vi "Experiment header-Overwrite values.vi"(10 "All header parameters in":T1={"LOGIN"={"User"="", "Profile"="", "Software Version"="", "Experiment Date Time"=timestamp(0 s since 1904-01-01)}, "GLOBAL PARAMETERS"={"MicroscopeID"="", "Microscope Type"="", "Objective"="", "Field of View (um)"=0.0, "Fill time (us)"=0.0, "Experiment Type"=enum."In vivo", "Stimuli Trigger"=FALSE, "Speed Logging"=FALSE}, "IMAGING MODES"={"Time Series"=FALSE, "Motor Zstack"=FALSE, "AOL Zstack"=FALSE, "Functional Imaging"=FALSE, "Volume Imaging"=FALSE}, "TIME SERIES"={"Basic Image meta data"={"Wavelength (nm)"=0.0, "# averaged frames"=0.0, "laser power (%)"=0.0, "Pockels"=0.0, "pixel dwell time (us)"=0.0, "pmt 1"=0.0, "pmt 2"=0.0, "back apperture"=0.0, "zoom"=0.0, "field of view"=0.0, "Frame Size"=0, "AOL x centre"=0.0, "AOL y centre"=0.0, "Stage x position"=0.0, "Stage y position"=0.0, "Stage z position"=0.0}, "AOL z"=0.0}, "MOTOR Z-STACK "={"Hdr Basic Image meta data"={"Wavelength (nm)"=0.0, "# averaged frames"=0.0, "laser power (%)"=0.0, "Pockels"=0.0, "pixel dwell time (us)"=0.0, "pmt 1"=0.0, "pmt 2"=0.0, "back apperture"=0.0, "zoom"=0.0, "field of view"=0.0, "Frame Size"=0, "AOL x centre"=0.0, "AOL y centre"=0.0, "Stage x position"=0.0, "Stage y position"=0.0, "Stage z position"=0.0}, "Z Start"=0.0, "Z Stop"=0.0, "No of Planes"=0, "Laser Power (%) at Z Start"=0.0, "Laser Power (%) at Z Stop"=0.0}, "AOL Z-STACK"={"Hdr Basic Image meta data"={"Wavelength (nm)"=0.0, "# averaged frames"=0.0, "laser power (%)"=0.0, "Pockels"=0.0, "pixel dwell time (us)"=0.0, "pmt 1"=0.0, "pmt 2"=0.0, "back apperture"=0.0, "zoom"=0.0, "field of view"=0.0, "Frame Size"=0, "AOL x centre"=0.0, "AOL y centre"=0.0, "Stage x position"=0.0, "Stage y position"=0.0, "Stage z position"=0.0}, "Z Start"=0.0, "Z Stop"=0.0, "No of Planes"=0, "Laser Power (%) at Z Start"=0.0, "Laser Power (%) at Z Stop"=0.0}, "FUNCTIONAL IMAGING"={"Functional Mode"=enum."Point", "Variable Length"=FALSE, "Variable Resolution"=FALSE, "Pockels Modulation"=FALSE, "Stimuli Trigger"=FALSE, "Cool down enabled"=FALSE, "AOL Mode"=enum."Raster", "Plane Mode"=0, "Miniscan Dwell time per pixel (us)"=0.0, "poi dwell time"=0.0, "Number of trials"=0.0, "Number of cycles"=0.0, "Number of pois"=0.0, "Number of miniscans"=0.0, "Number of pixels in miniscan"=0.0, "Rectangle ROI length"=0.0, "Rectangle ROI height"=0.0, "Frame rate (fps)"=0.0, "Acquisition Length"=0.0, "video length (sec)"=0.0, "Stimuli delay (sec)"=0.0, "Cool down time (sec)"=0.0, "Basic Image meta data"={"Wavelength (nm)"=0.0, "# averaged frames"=0.0, "laser power (%)"=0.0, "Pockels"=0.0, "pixel dwell time (us)"=0.0, "pmt 1"=0.0, "pmt 2"=0.0, "back apperture"=0.0, "zoom"=0.0, "field of view"=0.0, "Frame Size"=0, "AOL x centre"=0.0, "AOL y centre"=0.0, "Stage x position"=0.0, "Stage y position"=0.0, "Stage z position"=0.0}, "Z Start (um)"=0.0, "Z Stop (um)"=0.0}, "VOLUME IMAGING"={"Functional Mode"=enum."Point", "Variable Length"=FALSE, "Variable Resolution"=FALSE, "Pockels Modulation"=FALSE, "Stimuli Trigger"=FALSE, "Cool down enabled"=FALSE, "AOL Mode"=enum."Raster", "Plane Mode"=0, "Miniscan Dwell time per pixel (us)"=0.0, "poi dwell time"=0.0, "Number of trials"=0.0, "Number of cycles"=0.0, "Number of pois"=0.0, "Number of miniscans"=0.0, "Number of pixels in miniscan"=0.0, "Rectangle ROI length"=0.0, "Rectangle ROI height"=0.0, "Frame rate (fps)"=0.0, "Acquisition Length"=0.0, "video length (sec)"=0.0, "Stimuli delay (sec)"=0.0, "Cool down time (sec)"=0.0, "Basic Image meta data"={"Wavelength (nm)"=0.0, "# averaged frames"=0.0, "laser power (%)"=0.0, "Pockels"=0.0, "pixel dwell time (us)"=0.0, "pmt 1"=0.0, "pmt 2"=0.0, "back apperture"=0.0, "zoom"=0.0, "field of view"=0.0, "Frame Size"=0, "AOL x centre"=0.0, "AOL y centre"=0.0, "Stage x position"=0.0, "Stage y position"=0.0, "Stage z position"=0.0}, "Z Start (um)"=0.0, "Z Stop (um)"=0.0}, "MOVEMENT CORRECTION"={"Movement Correction"=FALSE, "Axial Reference"=FALSE, "Reference Source"=enum."Green channel", "Full Frame Size"=0.0, "Reference Field of View"=0.0, "Reference Zoom"=0.0, "Reference dwell time (us)"=0.0, "Reference X Pixels"=0.0, "Reference Y Pixels"=0.0, "Number of Z lines"=0.0, "Size of Z pixels"=0.0, "Axial Pixels"=0.0, "Ignore Z lines"=0.0, "Reference Scan Cycles"=0.0, "Reference Threshold XY"=0.0, "Reference Threshold Z"=0.0, "Reference Average XY"=0.0, "Reference Average Z"=0.0, "Proportional Scale"=0.0, "Integral Scale"=0.0, "Proportional Scale Z"=0.0, "Integral Scale Z"=0.0, "Diff Threshold"=0.0, "Diff Threshold Z"=0.0, "Sliding Average"=FALSE, "Reference count reset enabled"=FALSE, "Scan Interval (ms)"=0.0, "Ref Plot Refresh Rate (ms)"=0.0}, "CALIBRATION"={"Pockels Calibration File"=path "", "Calibration_ini file"=path "", "Setup_ini file"=path ""}, "STATISTICS"={"Z-stack duration (sec)"=0.0, "Number of acquired data-points"=0.0, "Acquisition time (ms)"=0.0, "Number of acquired frames"=0.0, "Intertrial times"=[]}, "BIOLOGY INFORMATION"={"Animal Code or Name"="", "Animal DoB"="", "Animal Age"="", "Animal Sex"="", "Animal Weight"="", "Date of Injection"="", "Date of Implant"="", "Site of Injection"="", "Animal Ear Notch"="", "AAV constructs"="", "Genetic background"="", "Optical reporter"="", "Region of brain imaged"="", "Other \ncomments"=""}, "Calibration Data"={"Objective Name"="", "Calibration Wavelength"=0.0, "Sum X"=0.0, "Sum Y"=0.0, "Diff X"=0.0, "Diff Y"=0.0, "Distortion Correction"=0.0, " Z norm to um Scaling"=0.0, " X norm to um Scaling"=0.0}, "Parameter Sweep Settings"={"Parameter Sweep Steps"={"MB Sep Start"=0.0, "MB Sep Stop"=0.25, "MB Sep Step"=1.0}, "Parameter Sweep"=enum."Dwell Time [us]", "# Sw. Planes"=0, "Basic image meta-data"={"Wavelength (nm)"=0.0, "# averaged frames"=0.0, "laser power (%)"=0.0, "Pockels"=0.0, "pixel dwell time (us)"=0.0, "pmt 1"=0.0, "pmt 2"=0.0, "back apperture"=0.0, "zoom"=0.0, "field of view"=0.0, "Frame Size"=200, "AOL x centre"=0.0, "AOL y centre"=0.0, "Stage x position"=0.0, "Stage y position"=0.0, "Stage z position"=0.0}}} {"Parameter Sweep Settings"."Basic image meta-data"."Frame Size" items=["100X100"=100, "128X128"=128, "200X200"=200, "256X256"=256, "512X512"=512, "1024x1024"=1024, "2048x2048"=2048]; "VOLUME IMAGING"."Plane Mode" items=["XY Plane", "XZ Plane", "YZ Plane", "arbitraryplane"]; "VOLUME IMAGING"."Basic Image meta data"."Frame Size" items=["100X100"=100, "128X128"=128, "200X200"=200, "256X256"=256, "512X512"=512, "1024x1024"=1024, "2048x2048"=2048]; "AOL Z-STACK"."Hdr Basic Image meta data"."Frame Size" items=["100X100"=100, "128X128"=128, "200X200"=200, "256X256"=256, "512X512"=512, "1024x1024"=1024, "2048x2048"=2048]; "MOTOR Z-STACK"."Hdr Basic Image meta data"."Frame Size" items=["100X100"=100, "128X128"=128, "200X200"=200, "256X256"=256, "512X512"=512, "1024x1024"=1024, "2048x2048"=2048]; "FUNCTIONAL IMAGING"."Plane Mode" items=["XY Plane", "XZ Plane", "YZ Plane", "arbitraryplane"]; "FUNCTIONAL IMAGING"."Basic Image meta data"."Frame Size" items=["100X100"=100, "128X128"=128, "200X200"=200, "256X256"=256, "512X512"=512, "1024x1024"=1024, "2048x2048"=2048]; "TIME SERIES"."Basic Image meta data"."Frame Size" items=["100X100"=100, "128X128"=128, "200X200"=200, "256X256"=256, "512X512"=512, "1024x1024"=1024, "2048x2048"=2048]}) -> (2 "All header parameters (FOV converted to um)":T1={"LOGIN"={"User"="", "Profile"="", "Software Version"="", "Experiment Date Time"=timestamp(0 s since 1904-01-01)}, "GLOBAL PARAMETERS"={"MicroscopeID"="", "Microscope Type"="", "Objective"="", "Field of View (um)"=0.0, "Fill time (us)"=0.0, "Experiment Type"=enum."In vivo", "Stimuli Trigger"=FALSE, "Speed Logging"=FALSE}, "IMAGING MODES"={"Time Series"=FALSE, "Motor Zstack"=FALSE, "AOL Zstack"=FALSE, "Functional Imaging"=FALSE, "Volume Imaging"=FALSE}, "TIME SERIES"={"Basic Image meta data"={"Wavelength (nm)"=0.0, "# averaged frames"=0.0, "laser power (%)"=0.0, "Pockels"=0.0, "pixel dwell time (us)"=0.0, "pmt 1"=0.0, "pmt 2"=0.0, "back apperture"=0.0, "zoom"=0.0, "field of view"=0.0, "Frame Size"=0, "AOL x centre"=0.0, "AOL y centre"=0.0, "Stage x position"=0.0, "Stage y position"=0.0, "Stage z position"=0.0}, "AOL z"=0.0}, "MOTOR Z-STACK "={"Hdr Basic Image meta data"={"Wavelength (nm)"=0.0, "# averaged frames"=0.0, "laser power (%)"=0.0, "Pockels"=0.0, "pixel dwell time (us)"=0.0, "pmt 1"=0.0, "pmt 2"=0.0, "back apperture"=0.0, "zoom"=0.0, "field of view"=0.0, "Frame Size"=0, "AOL x centre"=0.0, "AOL y centre"=0.0, "Stage x position"=0.0, "Stage y position"=0.0, "Stage z position"=0.0}, "Z Start"=0.0, "Z Stop"=0.0, "No of Planes"=0, "Laser Power (%) at Z Start"=0.0, "Laser Power (%) at Z Stop"=0.0}, "AOL Z-STACK"={"Hdr Basic Image meta data"={"Wavelength (nm)"=0.0, "# averaged frames"=0.0, "laser power (%)"=0.0, "Pockels"=0.0, "pixel dwell time (us)"=0.0, "pmt 1"=0.0, "pmt 2"=0.0, "back apperture"=0.0, "zoom"=0.0, "field of view"=0.0, "Frame Size"=0, "AOL x centre"=0.0, "AOL y centre"=0.0, "Stage x position"=0.0, "Stage y position"=0.0, "Stage z position"=0.0}, "Z Start"=0.0, "Z Stop"=0.0, "No of Planes"=0, "Laser Power (%) at Z Start"=0.0, "Laser Power (%) at Z Stop"=0.0}, "FUNCTIONAL IMAGING"={"Functional Mode"=enum."Point", "Variable Length"=FALSE, "Variable Resolution"=FALSE, "Pockels Modulation"=FALSE, "Stimuli Trigger"=FALSE, "Cool down enabled"=FALSE, "AOL Mode"=enum."Raster", "Plane Mode"=0, "Miniscan Dwell time per pixel (us)"=0.0, "poi dwell time"=0.0, "Number of trials"=0.0, "Number of cycles"=0.0, "Number of pois"=0.0, "Number of miniscans"=0.0, "Number of pixels in miniscan"=0.0, "Rectangle ROI length"=0.0, "Rectangle ROI height"=0.0, "Frame rate (fps)"=0.0, "Acquisition Length"=0.0, "video length (sec)"=0.0, "Stimuli delay (sec)"=0.0, "Cool down time (sec)"=0.0, "Basic Image meta data"={"Wavelength (nm)"=0.0, "# averaged frames"=0.0, "laser power (%)"=0.0, "Pockels"=0.0, "pixel dwell time (us)"=0.0, "pmt 1"=0.0, "pmt 2"=0.0, "back apperture"=0.0, "zoom"=0.0, "field of view"=0.0, "Frame Size"=0, "AOL x centre"=0.0, "AOL y centre"=0.0, "Stage x position"=0.0, "Stage y position"=0.0, "Stage z position"=0.0}, "Z Start (um)"=0.0, "Z Stop (um)"=0.0}, "VOLUME IMAGING"={"Functional Mode"=enum."Point", "Variable Length"=FALSE, "Variable Resolution"=FALSE, "Pockels Modulation"=FALSE, "Stimuli Trigger"=FALSE, "Cool down enabled"=FALSE, "AOL Mode"=enum."Raster", "Plane Mode"=0, "Miniscan Dwell time per pixel (us)"=0.0, "poi dwell time"=0.0, "Number of trials"=0.0, "Number of cycles"=0.0, "Number of pois"=0.0, "Number of miniscans"=0.0, "Number of pixels in miniscan"=0.0, "Rectangle ROI length"=0.0, "Rectangle ROI height"=0.0, "Frame rate (fps)"=0.0, "Acquisition Length"=0.0, "video length (sec)"=0.0, "Stimuli delay (sec)"=0.0, "Cool down time (sec)"=0.0, "Basic Image meta data"={"Wavelength (nm)"=0.0, "# averaged frames"=0.0, "laser power (%)"=0.0, "Pockels"=0.0, "pixel dwell time (us)"=0.0, "pmt 1"=0.0, "pmt 2"=0.0, "back apperture"=0.0, "zoom"=0.0, "field of view"=0.0, "Frame Size"=0, "AOL x centre"=0.0, "AOL y centre"=0.0, "Stage x position"=0.0, "Stage y position"=0.0, "Stage z position"=0.0}, "Z Start (um)"=0.0, "Z Stop (um)"=0.0}, "MOVEMENT CORRECTION"={"Movement Correction"=FALSE, "Axial Reference"=FALSE, "Reference Source"=enum."Green channel", "Full Frame Size"=0.0, "Reference Field of View"=0.0, "Reference Zoom"=0.0, "Reference dwell time (us)"=0.0, "Reference X Pixels"=0.0, "Reference Y Pixels"=0.0, "Number of Z lines"=0.0, "Size of Z pixels"=0.0, "Axial Pixels"=0.0, "Ignore Z lines"=0.0, "Reference Scan Cycles"=0.0, "Reference Threshold XY"=0.0, "Reference Threshold Z"=0.0, "Reference Average XY"=0.0, "Reference Average Z"=0.0, "Proportional Scale"=0.0, "Integral Scale"=0.0, "Proportional Scale Z"=0.0, "Integral Scale Z"=0.0, "Diff Threshold"=0.0, "Diff Threshold Z"=0.0, "Sliding Average"=FALSE, "Reference count reset enabled"=FALSE, "Scan Interval (ms)"=0.0, "Ref Plot Refresh Rate (ms)"=0.0}, "CALIBRATION"={"Pockels Calibration File"=path "", "Calibration_ini file"=path "", "Setup_ini file"=path ""}, "STATISTICS"={"Z-stack duration (sec)"=0.0, "Number of acquired data-points"=0.0, "Acquisition time (ms)"=0.0, "Number of acquired frames"=0.0, "Intertrial times"=[]}, "BIOLOGY INFORMATION"={"Animal Code or Name"="", "Animal DoB"="", "Animal Age"="", "Animal Sex"="", "Animal Weight"="", "Date of Injection"="", "Date of Implant"="", "Site of Injection"="", "Animal Ear Notch"="", "AAV constructs"="", "Genetic background"="", "Optical reporter"="", "Region of brain imaged"="", "Other \ncomments"=""}, "Calibration Data"={"Objective Name"="", "Calibration Wavelength"=0.0, "Sum X"=0.0, "Sum Y"=0.0, "Diff X"=0.0, "Diff Y"=0.0, "Distortion Correction"=0.0, " Z norm to um Scaling"=0.0, " X norm to um Scaling"=0.0}, "Parameter Sweep Settings"={"Parameter Sweep Steps"={"MB Sep Start"=0.0, "MB Sep Stop"=0.25, "MB Sep Step"=1.0}, "Parameter Sweep"=enum."Dwell Time [us]", "# Sw. Planes"=0, "Basic image meta-data"={"Wavelength (nm)"=0.0, "# averaged frames"=0.0, "laser power (%)"=0.0, "Pockels"=0.0, "pixel dwell time (us)"=0.0, "pmt 1"=0.0, "pmt 2"=0.0, "back apperture"=0.0, "zoom"=0.0, "field of view"=0.0, "Frame Size"=200, "AOL x centre"=0.0, "AOL y centre"=0.0, "Stage x position"=0.0, "Stage y position"=0.0, "Stage z position"=0.0}}} {"Parameter Sweep Settings"."Basic image meta-data"."Frame Size" items=["100X100"=100, "128X128"=128, "200X200"=200, "256X256"=256, "512X512"=512, "1024x1024"=1024, "2048x2048"=2048]; "VOLUME IMAGING"."Plane Mode" items=["XY Plane", "XZ Plane", "YZ Plane", "arbitraryplane"]; "VOLUME IMAGING"."Basic Image meta data"."Frame Size" items=["100X100"=100, "128X128"=128, "200X200"=200, "256X256"=256, "512X512"=512, "1024x1024"=1024, "2048x2048"=2048]; "AOL Z-STACK"."Hdr Basic Image meta data"."Frame Size" items=["100X100"=100, "128X128"=128, "200X200"=200, "256X256"=256, "512X512"=512, "1024x1024"=1024, "2048x2048"=2048]; "MOTOR Z-STACK"."Hdr Basic Image meta data"."Frame Size" items=["100X100"=100, "128X128"=128, "200X200"=200, "256X256"=256, "512X512"=512, "1024x1024"=1024, "2048x2048"=2048]; "FUNCTIONAL IMAGING"."Plane Mode" items=["XY Plane", "XZ Plane", "YZ Plane", "arbitraryplane"]; "FUNCTIONAL IMAGING"."Basic Image meta data"."Frame Size" items=["100X100"=100, "128X128"=128, "200X200"=200, "256X256"=256, "512X512"=512, "1024x1024"=1024, "2048x2048"=2048]; "TIME SERIES"."Basic Image meta data"."Frame Size" items=["100X100"=100, "128X128"=128, "200X200"=200, "256X256"=256, "512X512"=512, "1024x1024"=1024, "2048x2048"=2048]}, 3 "Field of view (um)":dbl)   [LabVIEW 2020]
uses:
  Global Variables/gl_UI Ctrl Refs.vi
  Typedefs/Header subclusters/Header params -Login.ctl
  Misc/Experiment Type.ctl
  Typedefs/Header subclusters/Header params-Global Parameters.ctl
  Typedefs/Header subclusters/Header params-Imaging Modes.ctl
  Typedefs/Header subclusters/Header params-Basic image meta data.ctl
  Typedefs/Header subclusters/Header params-Time Series.ctl
  Typedefs/Header subclusters/Header params-Functional Imaging.ctl
  Typedefs/Reference source.ctl
  Typedefs/Header subclusters/Header params-Movement correction.ctl
  Typedefs/Header subclusters/Header params-Calibration Setup.ctl
  Typedefs/Header subclusters/Header params-statistics.ctl
  Misc/Biology Information.ctl
  Typedefs/Header subclusters/Header params-Motor Z-stack.ctl
  Typedefs/Header subclusters/Header params-AOL Z-stack.ctl
  Typedefs/Header parameters cluster-ALL.ctl
  Typedefs/Frame Size.ctl
  Typedefs/Functional Mode.ctl
  Typedefs/AOL modes.ctl
  Typedefs/Plane Mode.ctl
  Typedefs/Header subclusters/Header params-calibration data.ctl
  Typedefs/Parameter sweep modes.ctl
  Typedefs/Parameter Sweep Steps.ctl
  Typedefs/Header subclusters/Header params-Parameter Sweep.ctl
panel:
  in  "error in (no error)":errorcluster
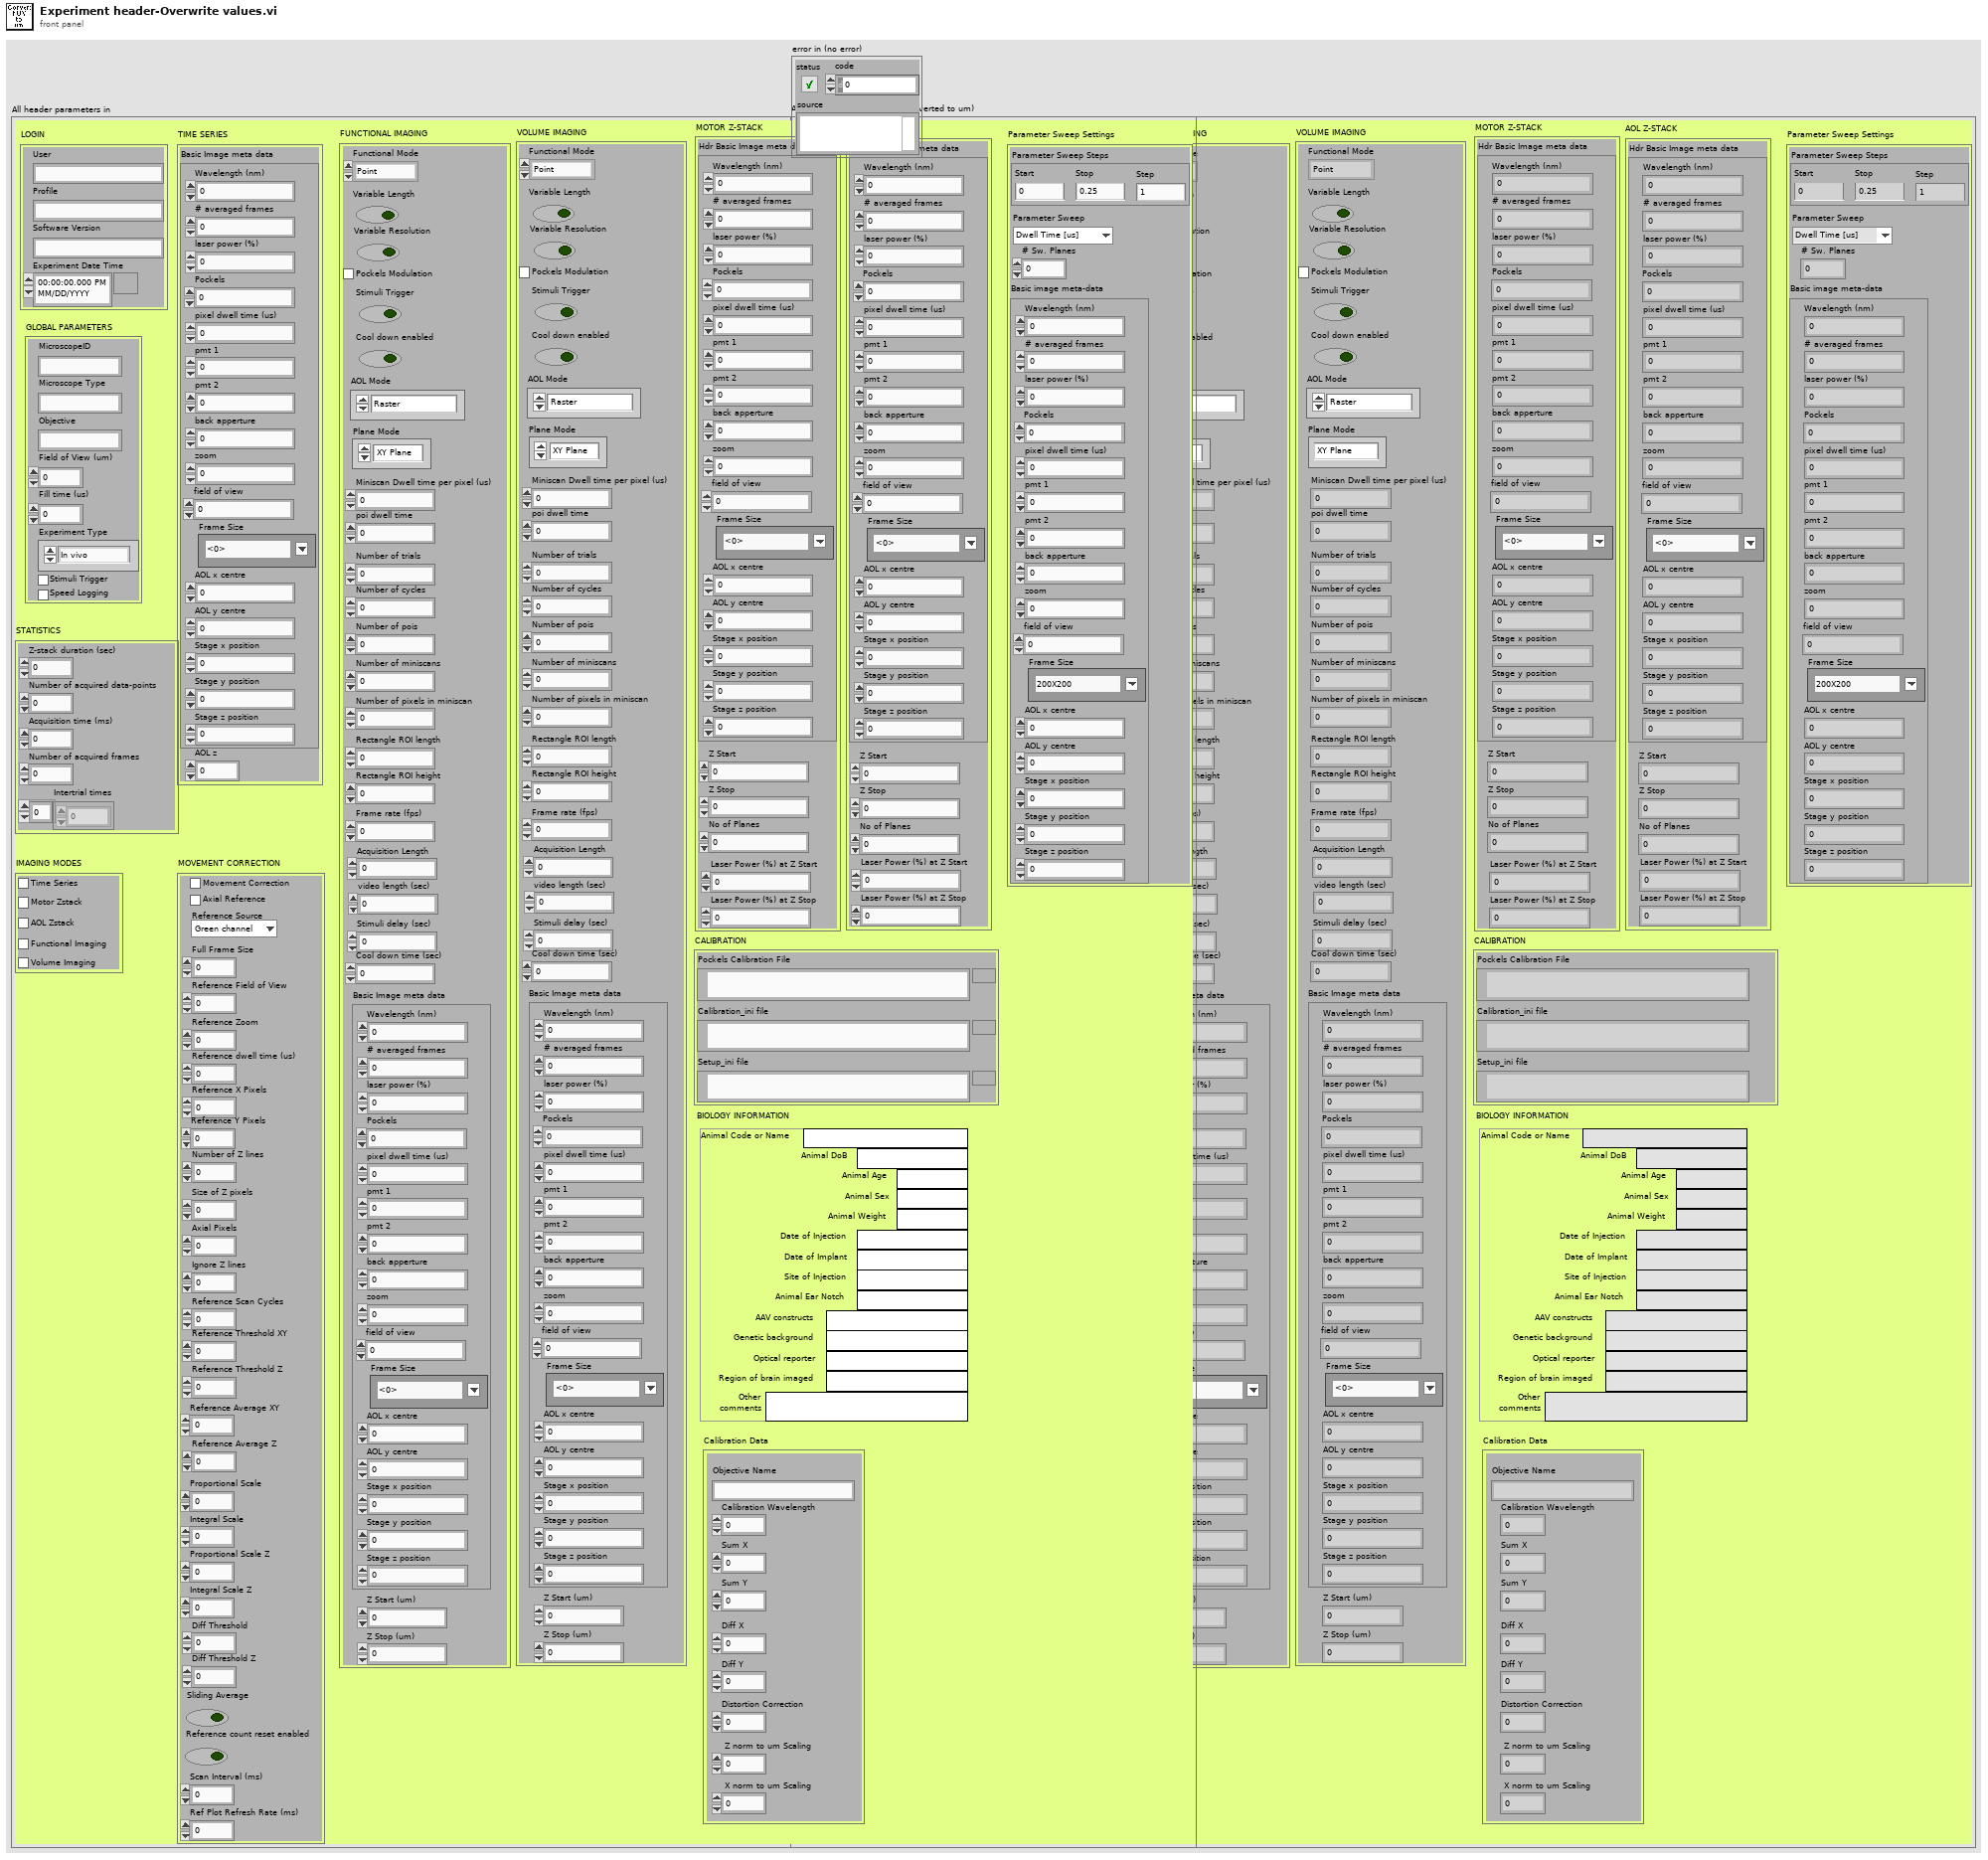
[diagram p1: front panel]
types:
  T1 = typedef "Header parameters cluster-ALL.ctl" = cluster{"LOGIN":T2, "GLOBAL PARAMETERS":T3, "IMAGING MODES":T5, "TIME SERIES":T6, "MOTOR Z-STACK ":T9, "AOL Z-STACK":T10, "FUNCTIONAL IMAGING":T11, "VOLUME IMAGING":T11, "MOVEMENT CORRECTION":T15, "CALIBRATION":T17, "STATISTICS":T18, "BIOLOGY INFORMATION":T19, "Calibration Data":T20, "Parameter Sweep Settings":T21}
  T2 = typedef "Header params -Login.ctl" = cluster{"User":string, "Profile":string, "Software Version":string, "Experiment Date Time":timestamp}
  T3 = typedef "Header params-Global Parameters.ctl" = cluster{"MicroscopeID":string, "Microscope Type":string, "Objective":string, "Field of View (um)":dbl, "Fill time (us)":dbl, "Experiment Type":T4, "Stimuli Trigger":bool, "Speed Logging":bool}
  T4 = typedef "Experiment Type.ctl" = enum16{"In vivo", "In vitro", "Testing", "Calibration", "Other"}
  T5 = typedef "Header params-Imaging Modes.ctl" = cluster{"Time Series":bool, "Motor Zstack":bool, "AOL Zstack":bool, "Functional Imaging":bool, "Volume Imaging":bool}
  T6 = typedef "Header params-Time Series.ctl" = cluster{"Basic Image meta data":T7, "AOL z":dbl}
  T7 = typedef "Header params-Basic image meta data.ctl" = cluster{"Wavelength (nm)":dbl, "# averaged frames":dbl, "laser power (%)":dbl, "Pockels":dbl, "pixel dwell time (us)":dbl, "pmt 1":dbl, "pmt 2":dbl, "back apperture":dbl, "zoom":dbl, "field of view":dbl, "Frame Size":T8, "AOL x centre":dbl, "AOL y centre":dbl, "Stage x position":dbl, "Stage y position":dbl, "Stage z position":dbl}
  T8 = typedef "Frame Size.ctl" = u16
  T9 = typedef "Header params-Motor Z-stack.ctl" = cluster{"Hdr Basic Image meta data":T7, "Z Start":dbl, "Z Stop":dbl, "No of Planes":i32, "Laser Power (%) at Z Start":dbl, "Laser Power (%) at Z Stop":dbl}
  T10 = typedef "Header params-AOL Z-stack.ctl" = cluster{"Hdr Basic Image meta data":T7, "Z Start":dbl, "Z Stop":dbl, "No of Planes":i32, "Laser Power (%) at Z Start":dbl, "Laser Power (%) at Z Stop":dbl}
  T11 = typedef "Header params-Functional Imaging.ctl" = cluster{"Functional Mode":T12, "Variable Length":bool, "Variable Resolution":bool, "Pockels Modulation":bool, "Stimuli Trigger":bool, "Cool down enabled":bool, "AOL Mode":T13, "Plane Mode":T14, "Miniscan Dwell time per pixel (us)":dbl, "poi dwell time":dbl, "Number of trials":dbl, "Number of cycles":dbl, "Number of pois":dbl, "Number of miniscans":dbl, "Number of pixels in miniscan":dbl, "Rectangle ROI length":dbl, "Rectangle ROI height":dbl, "Frame rate (fps)":dbl, "Acquisition Length":dbl, "video length (sec)":dbl, "Stimuli delay (sec)":dbl, "Cool down time (sec)":dbl, "Basic Image meta data":T7, "Z Start (um)":dbl, "Z Stop (um)":dbl}
  T12 = typedef "Functional Mode.ctl" = enum16{"Point", "Line", "Patch", "Plane", "Volume"}
  T13 = typedef "AOL modes.ctl" = enum16{"Raster", "Structural", "Pointing", "Mini Scan", "Alignment"}
  T14 = typedef "Plane Mode.ctl" = u16
  T15 = typedef "Header params-Movement correction.ctl" = cluster{"Movement Correction":bool, "Axial Reference":bool, "Reference Source":T16, "Full Frame Size":dbl, "Reference Field of View":dbl, "Reference Zoom":dbl, "Reference dwell time (us)":dbl, "Reference X Pixels":dbl, "Reference Y Pixels":dbl, "Number of Z lines":dbl, "Size of Z pixels":dbl, "Axial Pixels":dbl, "Ignore Z lines":dbl, "Reference Scan Cycles":dbl, "Reference Threshold XY":dbl, "Reference Threshold Z":dbl, "Reference Average XY":dbl, "Reference Average Z":dbl, "Proportional Scale":dbl, "Integral Scale":dbl, "Proportional Scale Z":dbl, "Integral Scale Z":dbl, "Diff Threshold":dbl, "Diff Threshold Z":dbl, "Sliding Average":bool, "Reference count reset enabled":bool, "Scan Interval (ms)":dbl, "Ref Plot Refresh Rate (ms)":dbl}
  T16 = typedef "Reference source.ctl" = enum16{"Green channel", "Red channel"}
  T17 = typedef "Header params-Calibration Setup.ctl" = cluster{"Pockels Calibration File":path, "Calibration_ini file":path, "Setup_ini file":path}
  T18 = typedef "Header params-statistics.ctl" = cluster{"Z-stack duration (sec)":dbl, "Number of acquired data-points":dbl, "Acquisition time (ms)":dbl, "Number of acquired frames":dbl, "Intertrial times":dbl[]}
  T19 = typedef "Biology Information.ctl" = cluster{"Animal Code or Name":string, "Animal DoB":string, "Animal Age":string, "Animal Sex":string, "Animal Weight":string, "Date of Injection":string, "Date of Implant":string, "Site of Injection":string, "Animal Ear Notch":string, "AAV constructs":string, "Genetic background":string, "Optical reporter":string, "Region of brain imaged":string, "Other \ncomments":string}
  T20 = typedef "Header params-calibration data.ctl" = cluster{"Objective Name":string, "Calibration Wavelength":dbl, "Sum X":dbl, "Sum Y":dbl, "Diff X":dbl, "Diff Y":dbl, "Distortion Correction":dbl, " Z norm to um Scaling":dbl, " X norm to um Scaling":dbl}
  T21 = typedef "Header params-Parameter Sweep.ctl" = cluster{"Parameter Sweep Steps":T22, "Parameter Sweep":T23, "# Sw. Planes":i32, "Basic image meta-data":T7}
  T22 = typedef "Parameter Sweep Steps.ctl" = cluster{"MB Sep Start":dbl, "MB Sep Stop":dbl, "MB Sep Step":dbl}
  T23 = typedef "Parameter sweep modes.ctl" = enum16{"None Selected", "Dwell Time [us]"}
  T24 = typedef "UI ctrl refs cluster.ctl" = cluster{"Top level VI path":path, "Top level VI ref":refnum<vi>, "User menu ref":refnum<k9>, "Sub Panel control":refnum<vi>, "Imaging Param Tab":refnum<vi>, "Occurrence-Start drivers":refnum<k4>, "Occurrence-Speed logging initialised":refnum<k4>, "Occurrence-XYZ stage initialised":refnum<k4>, "Exit button":refnum<vi>, "Status ind":refnum<vi>, "Set as origin":refnum<vi>, "Speed Logging":refnum<vi>, "Time Lapse":refnum<vi>, "Live Imaging":refnum<vi>, "AOL Z Stack":refnum<vi>, "Motor Z Stack":refnum<vi>, "Funct Acq button":refnum<vi>, "Hard Shutter":refnum<vi>, "Virtual Shutter":refnum<vi>, "Laser Power":refnum<vi>, "AOL Mode":refnum<vi>, "Frame Size":refnum<vi>, "Field of View":refnum<vi>, "Dwell Time":refnum<vi>, "Zoom":refnum<vi>, "AOL Z":refnum<vi>, "Objective":refnum<vi>, "Axis":refnum<vi>, "Paths & Names":refnum<vi>, "Experiment folder path (ind.)":refnum<vi>, "Last State (Ind.)":refnum<vi>, "Averages":refnum<vi>, "Angle (degrees)":refnum<vi>, "X centre":refnum<vi>, "Y centre":refnum<vi>, "Plane Mode":refnum<vi>, "# Planes":refnum<vi>, "Z Start":refnum<vi>, "Z Stop":refnum<vi>, "Z Step":refnum<vi>, "PMT 1":refnum<vi>, "PMT 2":refnum<vi>, "Stage XYZ Position":refnum<vi>, "Pockels@Z Start":refnum<vi>, "Pockels@Z Stop":refnum<vi>, "Obtain Z Start":refnum<vi>, "Obtain Z Stop":refnum<vi>, "Live stim.trig.period":refnum<vi>, "Live stim.trig.enable":refnum<vi>, "Movement Correction":refnum<vi>, "Load Reference Image":refnum<vi>, "XY Stage Move":refnum<vi>, "MovCor Cluster":refnum<vi>, "RefDAQParam":refnum<vi>, "Funct. Acq. Pockels Modulation":refnum<vi>, "Ref Laser Power":refnum<vi>, "Enable Video Recording":refnum<vi>, "Video Record-Live Imaging":refnum<vi>, "Video Record-Funct acq":refnum<vi>, "Reference Source":refnum<vi>, "AOL Z-stack Chirps Ready (ind)":refnum<vi>, "Target time between mov.cor. ref triggers (ms)":refnum<vi>, "Funct. Acq. Ref frame save":refnum<vi>, "Tracking button":refnum<vi>, "Show ref plots window":refnum<vi>, "Center freq ind (nm)":refnum<vi>, "Pickup mode (ind)":refnum<vi>, "Logging queue (ind)":refnum<vi>, "Back aperture power (ind.)":refnum<vi>, "Power after objective (ind.)":refnum<vi>, "Switch user":refnum<vi>, "Ls1 Conn. Status":refnum<vi>, "Ls1Tuning Status":refnum<vi>, "Ls1 Faults":refnum<vi>, "Ls1 Connection":refnum<vi>, "Ls1 Mode":refnum<vi>, "Ls1 POWER [mW]":refnum<vi>, "Ls1Shutter":refnum<vi>, "Ls1 Wavelength":refnum<vi>, "Ls1 Note":refnum<vi>, "Ls1 Confirm Wav":refnum<vi>, "Ls1 PreChrp Prism1":refnum<vi>, "Ls1 PreChrp Prism2":refnum<vi>, "Ls1 wav top Ind":refnum<vi>, "Ls1 power top Ind":refnum<vi>, "Ls1 Pump peak Hold":refnum<vi>, "Ls1 Status Ind":refnum<vi>, "Ls1 wav cancel":refnum<vi>, "Experiment Type":refnum<vi>, "Biology Information":refnum<vi>, "Camera recording status":refnum<vi>, "Parameter Sweep Steps":refnum<vi>, "Parameter Sweep":refnum<vi>, "Gen. Sweep Chirps":refnum<vi>, "Sweep Chirps ready":refnum<vi>, "# Sw. Planes":refnum<vi>, "Start Sweep":refnum<vi>, "Low-High Resolution Settings":refnum<vi>, "Optimise Obj. Pos.":refnum<vi>}
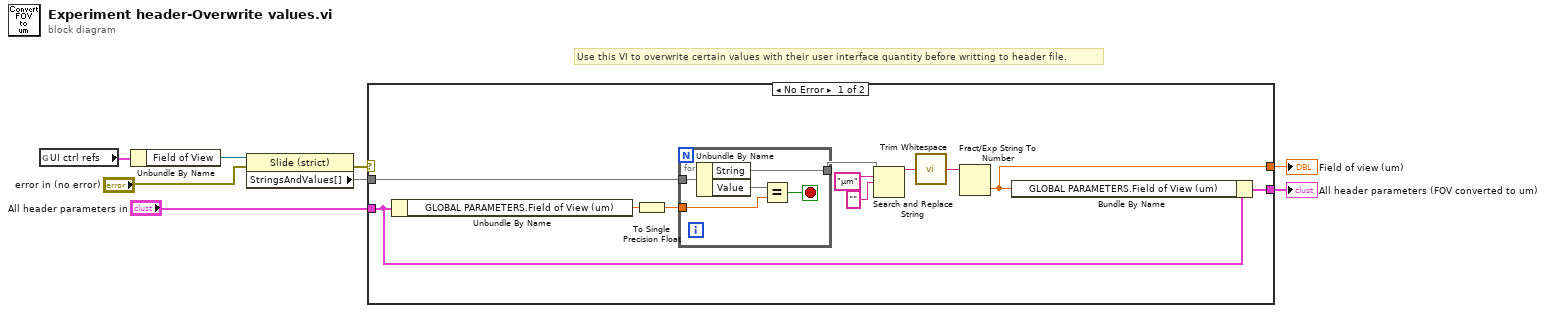
[diagram p0: block diagram]
diagram:
  # "Use this VI to overwrite certain values with their user interface quantity before writting to header file."
  n1 = global read "gl_UI Ctrl Refs.vi" "UI ctrl refs"() -> (w4:T24)
  n2 = Unbundle By Name(w4) -> ("Field of View"=w5:refnum<vi>)
  n3 = property on="Property Node" class="Slide (strict)"(reference=w5, error in="error in (no error)") -> (error out=w3:errorcluster, "StringsAndValues[]"=w6)  [unwired: 1 out]
  n4 = case shown="No Error" w3 {
    tunnel: [w19 w25] -> w8
    tunnel: [w9 _] -> w7
    tunnel: w6 -> [w13 _]
    tunnel: "All header parameters in" -> [w11 w25]
    frame No Error {
      n5 = Unbundle By Name(w11) -> ("GLOBAL PARAMETERS.Field of View (um)"=w10:dbl)
      n6 = To Single Precision Float(number=w10) -> (single precision float=w12:sgl)
      n7 = for {
        tunnel: w12 -> [w22]
        tunnel: w13 -> [w24]
        tunnel: [w20] -> w14
        stop <- w21 stop-if-true
        n8 = Unbundle By Name(w24) -> ("String"=w20, "Value"=w23)
        n9 = Equal?(x=w23, y=w22) -> (x = y?=w21:bool)
      }
      n10 = Search and Replace String(input string=w14, search string="µm", replace string="" ("replace string (\"\")")) -> (result string=w17:string)  [unwired: 5 in, 3 out]
      n11 = call <vilib>:"Trim Whitespace.vi"("string"=w17) -> ("trimmed string"=w18:string)  [unwired: 1 in]
      n12 = Fract/Exp String To Number(string=w18) -> (number=w9:dbl)  [unwired: 3 in, 1 out]
      n13 = Bundle By Name(cluster=w11, "GLOBAL PARAMETERS.Field of View (um)"=w9) -> (w19:T1)
    }
    frame Error {
      # "This case occurs when the time series viewer is not run through the main software. The error is effectively cleared and the FOV value is the input cluster is used."
    }
  }
  "Field of view (um)" <- w7
  "All header parameters (FOV converted to um)" <- w8
